vi "Read.vi"(8 "error in (no error)":errorcluster, 9 "timeout in ms (-1)":i32=-1, 11 "State in":refnum<class "State.lvclass">) -> (0 "error out":errorcluster, 1 "timed out?":bool, 2 "Value":variant)   [LabVIEW 2017, in "Promise Future.lvlib" / "State.lvclass"]
uses:
  State.lvclass
  State.lvclass/State.ctl
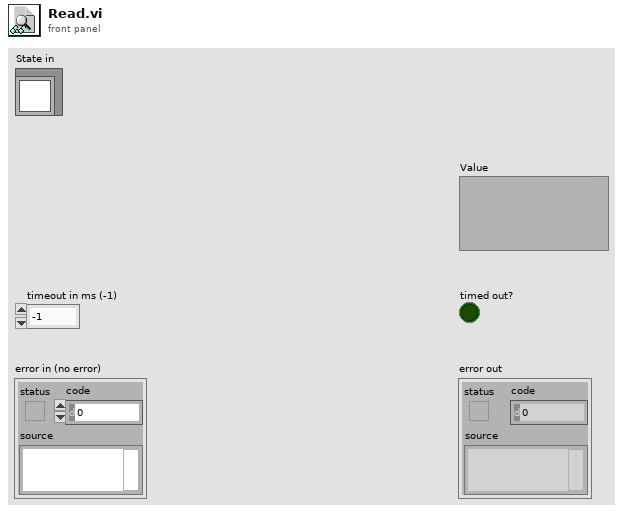
[diagram p1: front panel]
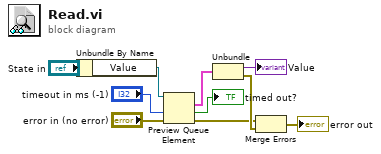
[diagram p0: block diagram]
diagram:
  n1 = Unbundle By Name("State in") -> ("Value"=w9:refnum<queue>)
  n2 = Preview Queue Element(queue=w9, timeout in ms (-1)="timeout in ms (-1)", error in (no error)="error in (no error)") -> (element=w8:cluster{"Value":variant, "Error":errorcluster}, timed out?=→"timed out?":bool, error out=w1:errorcluster)  [unwired: 1 out]
  n3 = Unbundle(w8) -> ("Value"=→"Value":variant, "Error"=w3:errorcluster)
  n4 = Merge Errors(w1, w3) -> (→"error out":errorcluster)
